vi "Cryomagnetics Control Panel.vi"(8 "error in (no error)":errorcluster, 11 "Class":refnum<class "Cryomagnetics Power Supply.lvclass">) -> (0 "error out":errorcluster, 3 "Cryomagnetics Power Supply out":refnum<class "Cryomagnetics Power Supply.lvclass">)   [LabVIEW 2015, in "Cryomagnetics Power Supply.lvclass"]
uses:
  Cryomagnetics Power Supply.lvclass
  Cryomagnetics Control Panel Data.ctl
  Sweep mode.ctl
panel:
  in  "Data":T1 {"Fast rate" format="%.4g"; "Low limit, kG" format="%.3g"; "High limit, kG" format="%.3g"; "Rates, A/s" format="%.4g"}
  # "Magnet Control"
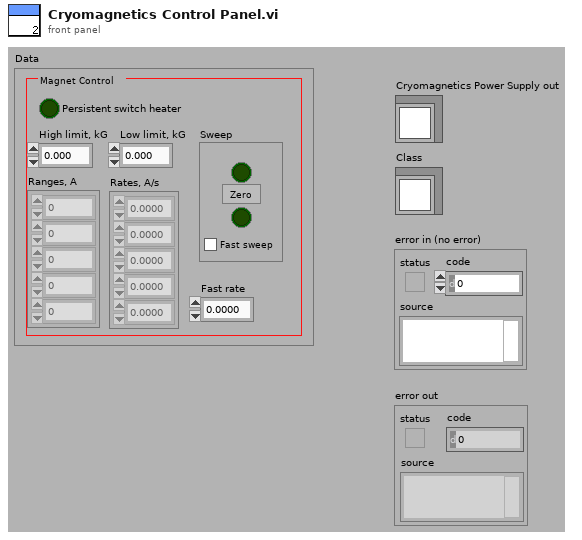
[diagram p1: front panel]
types:
  T1 = typedef "Cryomagnetics Control Panel Data.ctl" = cluster{"Persistent switch heater":bool, "Rates, A/s":dbl[], "Ranges, A":dbl[], "High limit, kG":dbl, "Low limit, kG":dbl, "Sweep ":T2, "Fast rate":dbl}
  T2 = typedef "Sweep mode.ctl" = cluster{"zero":bool, "sweep up":bool, "sweep down":bool, "fast sweep":bool}
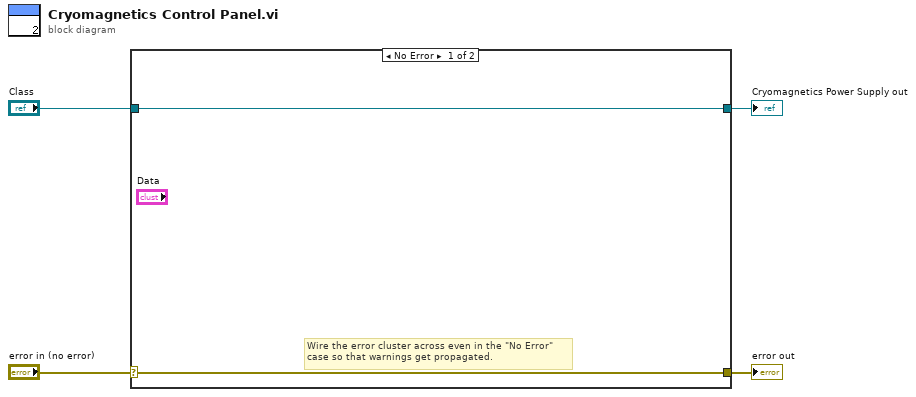
[diagram p0: block diagram]
diagram:
  n1 = case shown="No Error" "error in (no error)" {
    selector: "error in (no error)" -> [w5 w8]
    tunnel: [w5 w8] -> w3
    tunnel: [w6 w7] -> w1
    tunnel: "Class" -> [w6 w7]
    frame No Error {
      # "Wire the error cluster across even in the \"No Error\"\ncase so that warnings get propagated."
    }
    frame Error {
    }
  }
  "error out" <- w3
  "Cryomagnetics Power Supply out" <- w1
